vi "Format table.vi"(11 "Table输入":refnum<vi>) -> ()   [LabVIEW 2016, in "数据查询.lvlib"]
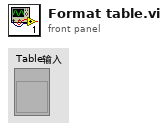
[diagram p1: front panel]
types:
  T1 = cluster{"Font Name:":string, "Size":i16, "Strikeout?":bool, "Italic?":bool, "Underline?":bool, "Outline?":bool, "Shadow?":bool, "Bold?":bool}
  T2 = typedef "LVFontTypeDef.ctl" = cluster{"Font Name":string, "Size":u16, "Bold":bool, "Italic":bool, "Underline":bool, "Strikeout":bool, "Color":u32}
  T3 = enum16{"User-specified Font", "Application Font", "System Font", "Dialog Font"}
  T4 = cluster{"left":i16, "top":i16, "right":i16, "bottom":i16}
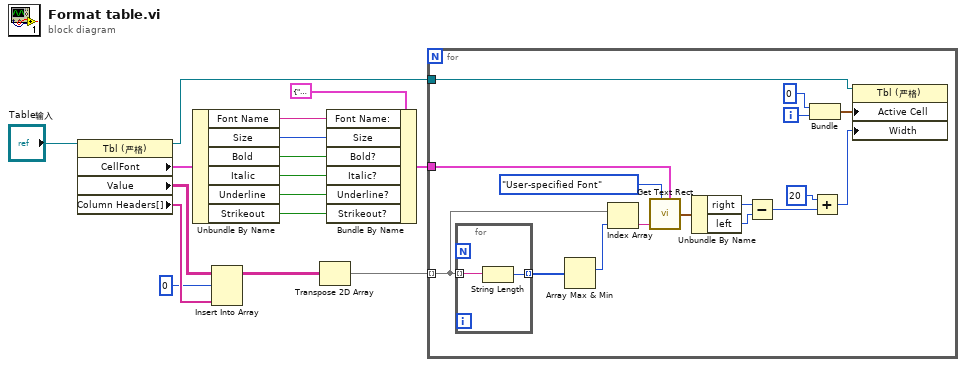
[diagram p0: block diagram]
diagram:
  n1 = property class="Tbl (严格)"(reference="Table输入") -> (reference out=w6:refnum<vi>, "CellFont"=w9:T2, "Value"=w3:string[][], "Column Headers[]"=w2:string[])  [unwired: 1 in, 1 out]
  n2 = Unbundle By Name(w9) -> ("Font Name"=w15:string, "Size"=w14:u16, "Bold"=w13:bool, "Italic"=w12:bool, "Underline"=w11:bool, "Strikeout"=w10:bool)
  n3 = Insert Into Array(array=w3, index (row)=0 ("索引 (行)"), new element=w2) -> (w4:string[][])  [unwired: 1 in]
  n4 = Transpose 2D Array(2D array=w4) -> (transposed array=w5:string[][])
  n5 = Bundle By Name(cluster=T1 {"Font Name:"="", "Size"=0, "Strikeout?"=FALSE, "Italic?"=FALSE, "Underline?"=FALSE, "Outline?"=FALSE, "Shadow?"=FALSE, "Bold?"=FALSE} ("[user-specified font]"), "Font Name:"=w15, "Size"=w14, "Bold?"=w13, "Italic?"=w12, "Underline?"=w11, "Strikeout?"=w10) -> (w7:T1)
  n6 = for {
    tunnel: w5 -> [w22] mode=indexing
    tunnel: w6 -> [w18]
    tunnel: w7 -> [w19]
    i -> [w32]
    n7 = for {
      tunnel: w22 -> [w34] mode=indexing
      tunnel: [w33] -> w21 mode=indexing
      n8 = String Length(string=w34) -> (length=w33:i32)
    }
    n9 = Array Max & Min(array=w21) -> (max index (indices)=w20:i32)  [unwired: 3 out]
    n10 = Index Array(array=w22, index=w20) -> (element=w23:string)
    n11 = call <vilib>:"Get Text Rect.vi"("desired font(Application)"=T3."User-specified Font", "text"=w23, "[user-specified font]"=w19) -> ("rect"=w26:T4)  [unwired: 6 in]
    n12 = Unbundle By Name(w26) -> ("right"=w25:i16, "left"=w24:i16)
    n13 = Subtract(x=w25, y=w24) -> (x-y=w17:i16)
    n14 = Bundle(0, w32) -> (w28:cluster{i32, i32})  [unwired: 1 in]
    n15 = Add(x=i16 20, y=w17) -> (x+y=w29:i16)
    n16 = property on="属性节点" class="Tbl (严格)"(reference=w18, "Active Cell"=w28, "Width"=w29) -> ()  [unwired: 1 in, 2 out]
  }
